vi "Vision Research Phantom Series PhCon PhGet String.vi"(0 "CN [in]":u32, 1 "Sel":T1 items=["gsHasMechanicalShutter"=1025, "gsHasBlackLevel4"=1027, "gsHasCardFlash"=1051, "gsHas10G"=2000, "gsSupportsInternalBlackRef"=1026, "gsSupportsImageTrig"=1040, "gsSupportsCardFlash"=1050, "gsSupportsMagazine"=8193, "gsSupportsHQMode"=8194, "gsSupportsGenlock"=8195, "gsSupportsEDR"=8196, "gsSupportsAutoExposure"=8197, "gsSupportsTurbo"=8198, "gsSupportsBurstMode"=8199, "gsSupportsShutterOff"=8200, "gsSupportsDualSDIOutput"=8201, "gsSupportsRecordingCines"=8202, "gsSupportsV444"=8203, "gsSupportsInterlacedSensor"=8204, "gsSupportsRampFRP"=8205, "gsSensorTemperature"=1028, "gsCameraTemperature"=1029, "gsThermoElectricPower"=1030, "gsSensorTemperatureThreshold"=1031, "gsCameraTemperatureThreshold"=1032, "gsVideoPlayCine"=1033, "gsVideoPlaySpeed"=1034, "gsVideoOutputConfig"=1035, "gsMechanicalShutter"=1036, "gsImageTrigThreshold"=1041, "gsImageTrigAreaPercentage"=1042, "gsImageTrigSpeed"=1043, "gsImageTrigMode"=1044, "gsImageTrigRect"=1045, "gsAutoProgress"=1046, "gsAutoBlackRef"=1047, "gsCardFlashSizeK"=1052, "gsCardFlashFreeK"=1053, "gsCardFlashError"=1054, "gsEthernetAddress"=1055, "gsEthernetMask"=1056, "gsEthernetBroadcast"=1057, "gsEthernetGateway"=1058, "gsLensFocus"=1059, "gsLensAperature"=1060, "gsLensAperatureRange"=1061, "gsLensDescription"=1062, "gsLensFocusInProgress"=1063, "gsLensFocusAtLimit"=1064, "gsGenlock"=1065, "gsGenlockStatus"=1066, "gsTurboMode"=1068, "gsModel"=1069, "gsIPAddress"=1070], 5 "Error In (no error)":errorcluster) -> (14 "CN [out]":u32=1, 15 "pVal [out]":string, 19 "Error Out":errorcluster)   [LabVIEW 2013, in "VRI.lvlib"]
doc: "PhGet\nHRESULT PhGet(UNIT CN, UINT Sel, PVOID pVal)\n\nParameters\nCN [in]\n Camera number.\nSel [in]\n Selection value indicating the information to be retrieved.\npVal [out]\n Pointer to the buffer in which the value for the requested property is to be returned.\n\nReturn Value\nThe function returns ERR_Ok in case of success or an error code, otherwise. To get extended error information call PhGetErrorMessage.\n\nRemarks\nThis function gets information about the given camera based on a selection code. For a complete list of currently available selectors, go to Appendix 2.\n\nRequired Header\nPhCon.h"
uses:
  VRI.lvlib
  _Type Defs/PhCon GS.ctl
  Phantom DLLs/PhCon.dll
panel:
  # "For instructions on the use of this VI, press Ctrl+H to display the help window and move the mouse over the icon, controls, and indicators"
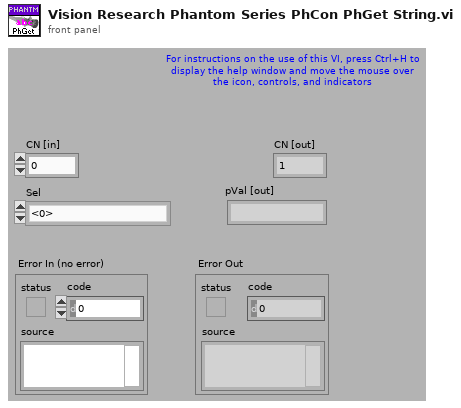
[diagram p1: front panel]
types:
  T1 = typedef "VRI.lvlib/PhCon GS.ctl" = u16
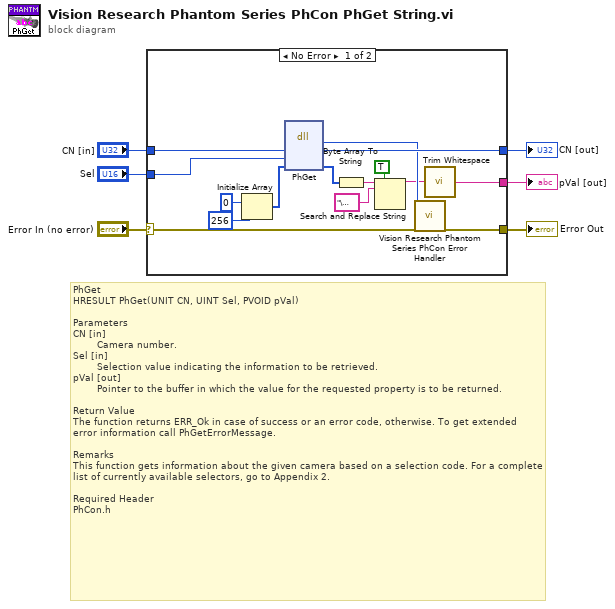
[diagram p0: block diagram]
diagram:
  # "PhGet\nHRESULT PhGet(UNIT CN, UINT Sel, PVOID pVal)\n\nParameters\nCN [in]\n\t       Camera number.\nSel [in]\n\t       Selection value indicating the information to be retrieved.\npVal [out]\n        Pointer to the buffer in which the value for the requested property is to be returned.\n\nReturn Value\nThe function returns ERR_Ok in case of success or an error code, otherwise. To get extended error information call PhGetErrorMessage.\n\nRemarks\nThis function gets information about the given camera based on a selection code. For a complete list of currently available selectors, go to Appendix 2.\n\nRequired Header\nPhCon.h"
  n1 = case shown="No Error" "Error In (no error)" {
    selector: "Error In (no error)" -> [w21 w23]
    tunnel: [w20 w23] -> w5
    tunnel: "CN [in]" -> [w19 w22]
    tunnel: [w18 w22] -> w3
    tunnel: "Sel" -> [w17 _]
    tunnel: [w16 _] -> w1
    frame No Error {
      n2 = Initialize Array(u8 0 ("element"), 256 ("dimension size")) -> (w11:u8[])
      n3 = dll-call lib="C:/Projects/SDK/32-bit/Vision Research Phantom Series Labview Driver/Phantom DLLs/PhCon.dll" fn="PhGet"("CN"=w19, "Sel"=w17, "pVal"=w11) -> ("HRESULT"=w15:i32, "CN"=w18:u32, "pVal"=w14:u8[])  [unwired: 3 in, 3 out]
      n4 = Byte Array To String(unsigned byte array=w14) -> (string=w8:string)
      n5 = Search and Replace String(replace all?=TRUE ("replace all? (F)"), input string=w8, search string="\u0000") -> (result string=w7:string)  [unwired: 5 in, 3 out]
      n6 = call "Vision Research Phantom Series PhCon Error Handler.vi"("ErrNo"=w15, "Error In (no error)"=w21) -> ("Error Out"=w20:errorcluster)  [unwired: 17 out]
      n7 = call <vilib>:"Trim Whitespace.vi"("string"=w7) -> ("trimmed string"=w16:string)  [unwired: 1 in]
    }
    frame Error {
    }
  }
  "Error Out" <- w5
  "CN [out]" <- w3
  "pVal [out]" <- w1
